vi "source_measure.vi"(8 "error in (no error)":errorcluster, 11 "Input parameters":T1={"Measurement type"=enum."Debug", "Sensor type"=enum."HPK_8in_271ch", "Identifier"="test.txt", "Open after execution?"=FALSE, "Plot after execution?"=FALSE, "Display channel"=0, "Voltage Delay (s)"=0.5, "Switch Delay (s)"=0.01, "VISA resource name source"="", "VISA resource name DMM"="", "VISA resource name LCR"="", "Compliance  Level (A)"=10.0, "Voltage Limit (V)"=1000.0, "Data storage location"="", "Scan voltages"="", "Use source as DMM?"=FALSE, "LCR signal frequenzy (Hz)"=10.0, "DMM device"=enum."Keithley2001", "Sampling number"=1, "Use env. sensors on"=enum."Sensirion sht1x/7x", "Switchboard Handle"=0, "Use Switchboard"=FALSE, "LCR signal voltage (V)"=10000.0, "Repeat"=1, "Scan voltages IV"="", "Scan voltages CV"="", "Hex pad numbers?"=FALSE, "Set measurement type"=enum."Debug", "Custom pad scan"="", "IV voltage Delay (s)"=0.5, "CV voltage Delay (s)"=0.5, "Needle measurement?"=FALSE, "Comments"="test.txt", "LCR signal frequenzy (kHz)"=10.0, "Compliance  Level (uA)"=10.0, "Open Correction Array"=array2304x3[6912 elements], "Current set voltage"=0.0, "Last set voltage"=0.0, "Current channel"=0, "Last OpenCorrection index"=-1, "Total curr/vltg every x steps"=10, "Current channel iteration"=0, "No CV corrections"=FALSE, "Mapfile"="", "Corrfile"="", "IV voltage file"=path "", "CV voltage file"=path "", "IV Switch Delay (s)"=0.01, "CV Switch Delay (s)"=0.01, "Invert polarity"=FALSE, "Set debug dirs"=FALSE, "Is n on p"=FALSE, "Source interlock?"=TRUE, "Voltage file used?"=FALSE, "Pad mask"="", "Mask pad above (uA)"=1.0, "LCR device"=enum."LCR_E4980", "Source device"=enum."Source_2410", "HexPlot binary path"="", "PadReductionFactor"=1.0, "Temperature degC"="", "Fluence [neq]"="", "Annealing [min]"=""} {"CV Switch Delay (s)" format="%#_13g"; "IV Switch Delay (s)" format="%#_13g"; "Last set voltage" format="%#_13g"; "Current set voltage" format="%#_13g"; "CV voltage Delay (s)" format="%#_13g"; "IV voltage Delay (s)" format="%#_13g"; "Voltage Limit (V)" format="%#_13g"; "Voltage Delay (s)" format="%#_13g"; "Switch Delay (s)" format="%#_13g"}) -> (0 "error out":errorcluster, 2 "Total current":dbl, 3 "Input parameters":T1={"Measurement type"=enum."Debug", "Sensor type"=enum."HPK_8in_271ch", "Identifier"="test.txt", "Open after execution?"=FALSE, "Plot after execution?"=FALSE, "Display channel"=0, "Voltage Delay (s)"=0.5, "Switch Delay (s)"=0.01, "VISA resource name source"="", "VISA resource name DMM"="", "VISA resource name LCR"="", "Compliance  Level (A)"=10.0, "Voltage Limit (V)"=1000.0, "Data storage location"="", "Scan voltages"="", "Use source as DMM?"=FALSE, "LCR signal frequenzy (Hz)"=10.0, "DMM device"=enum."Keithley2001", "Sampling number"=1, "Use env. sensors on"=enum."Sensirion sht1x/7x", "Switchboard Handle"=0, "Use Switchboard"=FALSE, "LCR signal voltage (V)"=10000.0, "Repeat"=1, "Scan voltages IV"="", "Scan voltages CV"="", "Hex pad numbers?"=FALSE, "Set measurement type"=enum."Debug", "Custom pad scan"="", "IV voltage Delay (s)"=0.5, "CV voltage Delay (s)"=0.5, "Needle measurement?"=FALSE, "Comments"="test.txt", "LCR signal frequenzy (kHz)"=10.0, "Compliance  Level (uA)"=10.0, "Open Correction Array"=array2304x3[6912 elements], "Current set voltage"=0.0, "Last set voltage"=0.0, "Current channel"=0, "Last OpenCorrection index"=-1, "Total curr/vltg every x steps"=10, "Current channel iteration"=0, "No CV corrections"=FALSE, "Mapfile"="", "Corrfile"="", "IV voltage file"=path "", "CV voltage file"=path "", "IV Switch Delay (s)"=0.01, "CV Switch Delay (s)"=0.01, "Invert polarity"=FALSE, "Set debug dirs"=FALSE, "Is n on p"=FALSE, "Source interlock?"=TRUE, "Voltage file used?"=FALSE, "Pad mask"="", "Mask pad above (uA)"=1.0, "LCR device"=enum."LCR_E4980", "Source device"=enum."Source_2410", "HexPlot binary path"="", "PadReductionFactor"=1.0, "Temperature degC"="", "Fluence [neq]"="", "Annealing [min]"=""} {"CV Switch Delay (s)" format="%#_13g"; "IV Switch Delay (s)" format="%#_13g"; "Last set voltage" format="%#_13g"; "Current set voltage" format="%#_13g"; "CV voltage Delay (s)" format="%#_13g"; "IV voltage Delay (s)" format="%#_13g"; "Voltage Limit (V)" format="%#_13g"; "Voltage Delay (s)" format="%#_13g"; "Switch Delay (s)" format="%#_13g"}, 4 "Compliance reached?":bool, 5 "Actual voltage":dbl)   [LabVIEW 2020]
doc: "Determines current voltage and current through source meter."
uses:
  <instrlib>/Keithley 24XX/Keithley 24XX.lvlib
  <instrlib>/Keithley 648X Series/Keithley 648X Series.lvlib
  input_params.ctl
panel:
  out "Effective resistance":sgl
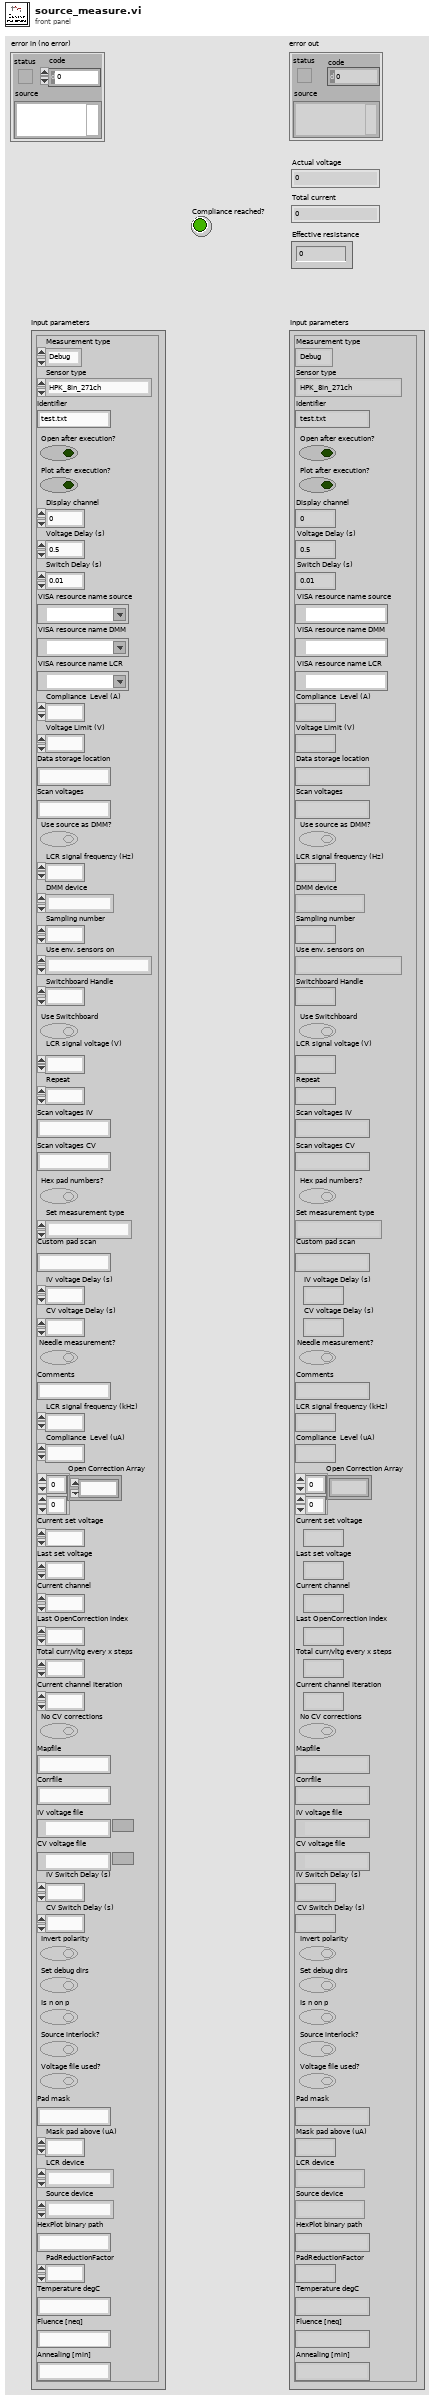
[diagram p1: front panel]
types:
  T1 = typedef "input_params.ctl" = cluster{"Measurement type":enum16{"IV", "CV", "Debug", "Test_contact"}, "Sensor type":enum16{"HPK_6in_135ch", "HPK_8in_271ch", "IFX_8in_256ch", "Diode", "HPK_6in_239ch", "Full_Matrix", "HPK_8in_271ch_full", "LumiCal", "HPK_8in_444ch", "HPK_8in_198ch_2019", "HPK_8in_MGW_LD_full", "HPK_8in_MGW_LD_a_type_top", "HPK_8in_MGW_LD_a_type_bottom", "HPK_8in_MGW_LD_b_type_left", "HPK_8in_MGW_LD_b_type_right", "HPK_8in_MGW_LD_c_type_left", "HPK_8in_MGW_LD_c_type_right", "HPK_8in_MGW_HD_full", "HPK_8in_MGW_HD_a_type_top", "HPK_8in_MGW_HD_a_type_bottom", "HPK_8in_MGW_HD_b_type_left", "HPK_8in_MGW_HD_b_type_right", "HPK_8in_MGW_HD_c_type_left", "HPK_8in_MGW_HD_c_type_right", "CALICE_6in_256ch"}, "Identifier":string, "Open after execution?":bool, "Plot after execution?":bool, "Display channel":i32, "Voltage Delay (s)":dbl, "Switch Delay (s)":dbl, "VISA resource name source":refnum<visa-resource-name>, "VISA resource name DMM":refnum<visa-resource-name>, "VISA resource name LCR":refnum<visa-resource-name>, "Compliance  Level (A)":dbl, "Voltage Limit (V)":dbl, "Data storage location":string, "Scan voltages":string, "Use source as DMM?":bool, "LCR signal frequenzy (Hz)":dbl, "DMM device":enum16{"Keithley2001", "Keithley2450", "Keithley2410", "Keithley6485", "Keithley6487", "Keithley6517"}, "Sampling number":i32, "Use env. sensors on":enum16{"Sensirion sht1x/7x", "Switch Matrix", "Probecard"}, "Switchboard Handle":u32, "Use Switchboard":bool, "LCR signal voltage (V)":dbl, "Repeat":i32, "Scan voltages IV":string, "Scan voltages CV":string, "Hex pad numbers?":bool, "Set measurement type":enum16{"IV", "CV", "Debug", "Test_contact", "IV+CV"}, "Custom pad scan":string, "IV voltage Delay (s)":dbl, "CV voltage Delay (s)":dbl, "Needle measurement?":bool, "Comments":string, "LCR signal frequenzy (kHz)":dbl, "Compliance  Level (uA)":dbl, "Open Correction Array":dbl[][], "Current set voltage":dbl, "Last set voltage":dbl, "Current channel":i32, "Last OpenCorrection index":i32, "Total curr/vltg every x steps":i32, "Current channel iteration":i32, "No CV corrections":bool, "Mapfile":string, "Corrfile":string, "IV voltage file":path, "CV voltage file":path, "IV Switch Delay (s)":dbl, "CV Switch Delay (s)":dbl, "Invert polarity":bool, "Set debug dirs":bool, "Is n on p":bool, "Source interlock?":bool, "Voltage file used?":bool, "Pad mask":string, "Mask pad above (uA)":dbl, "LCR device":enum16{"LCR_E4980", "AGILENT_4263X"}, "Source device":enum16{"Source_2410", "Source_6487"}, "HexPlot binary path":string, "PadReductionFactor":dbl, "Temperature degC":string, "Fluence [neq]":string, "Annealing [min]":string}
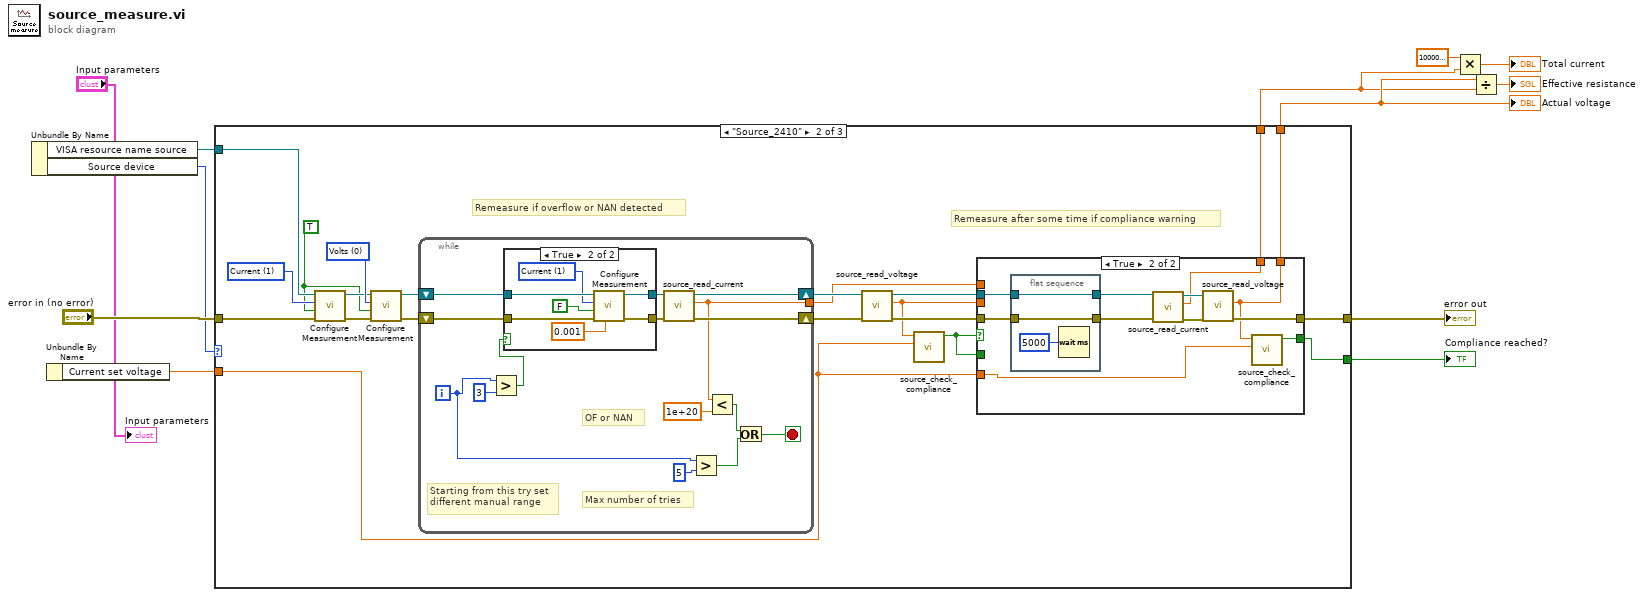
[diagram p0: block diagram]
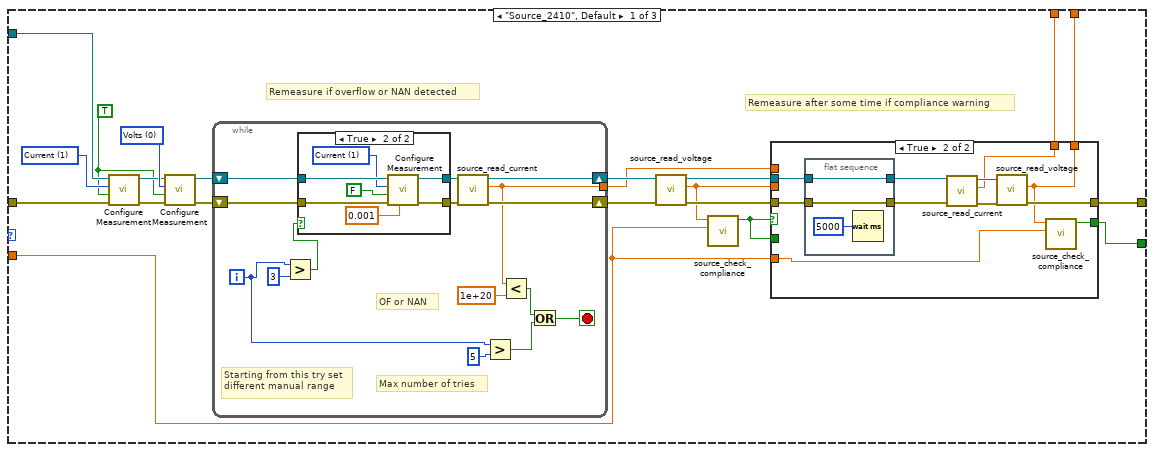
[diagram p2: hidden frame]
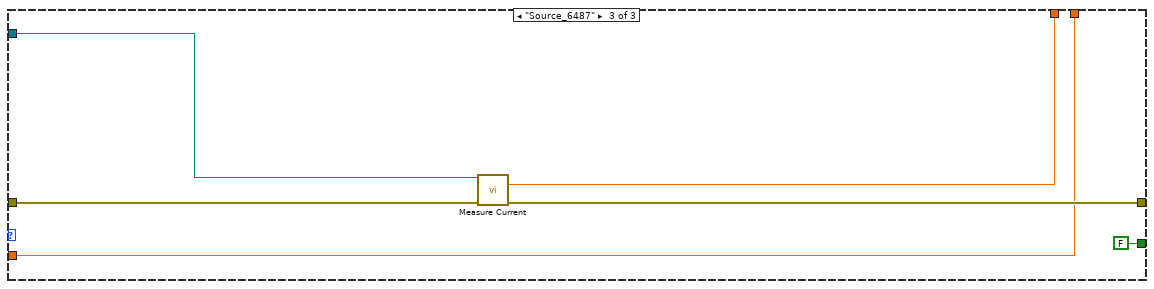
[diagram p7: hidden frame]
diagram:
  n1 = Unbundle By Name("Input parameters") -> ("VISA resource name source"=w12:refnum<visa-resource-name>, "Source device"=w1:enum16{"Source_2410", "Source_6487"})
  n2 = Unbundle By Name("Input parameters") -> ("Current set voltage"=w2:dbl)
  n3 = case shown="\"Source_2470\"" w1 {
    tunnel: w12 -> [w33 w96 w140]
    tunnel: "error in (no error)" -> [w32 w95 w139]
    tunnel: [w21 w84 w143] -> w6
    tunnel: [w19 w82 FALSE ("Is compliance?")] -> w5
    tunnel: [w17 w80 w141] -> w4
    tunnel: [w16 w79 w142] -> w3
    tunnel: w2 -> [w14 w77 w141]
    frame "Source_2410", Default {
      w27 = TRUE
      w30 = u16 0 items=["Volts", "Current", "Resistance"] ("Function (0: Volts)")
      w31 = u16 1 items=["Volts", "Current", "Resistance"] ("Function (0: Volts)")
      # "Remeasure after some time if compliance warning"
      # "Remeasure if overflow or NAN detected"
      n4 = call <instrlib>:"Configure Measurement.vi"("error in (no error)"=w32, "Enable Auto Range (T:Enable)"=w27, "Function (0: Volts)"=w31, "VISA resource name"=w33) -> ("error out"=w29:errorcluster, "VISA resource name out"=w28:refnum<visa-resource-name>)  [unwired: 6 in]
      n5 = call <instrlib>:"Configure Measurement.vi"("error in (no error)"=w29, "Enable Auto Range (T:Enable)"=w27, "Function (0: Volts)"=w30, "VISA resource name"=w28) -> ("error out"=w26:errorcluster, "VISA resource name out"=w25:refnum<visa-resource-name>)  [unwired: 6 in]
      n6 = while {
        tunnel: [w44] -> w13
        shift-right: [w48] -> w24
        shift-left: w26 -> [w38]
        shift-right: [w47] -> w23
        shift-left: w25 -> [w36]
        i -> [w40]
        stop <- w41 stop-if-true
        # "Starting from this try set\ndifferent manual range"
        # "OF or NAN"
        # "Max number of tries"
        n7 = Greater?(x=w40, y=3) -> (0:w34:bool)
        n8 = case shown="True" w34 {
          tunnel: w38 -> [w49 w57]
          tunnel: [w49 w56] -> w37
          tunnel: w36 -> [w50 w55]
          tunnel: [w50 w54] -> w35
          frame False {
          }
          frame True {
            w53 = u16 1 items=["Volts", "Current", "Resistance"] ("Function (0: Volts)")
            n9 = call <instrlib>:"Configure Measurement.vi"("Manual Range (1.0)"=0.001, "error in (no error)"=w57, "Enable Auto Range (T:Enable)"=FALSE, "Function (0: Volts)"=w53, "VISA resource name"=w55) -> ("error out"=w56:errorcluster, "VISA resource name out"=w54:refnum<visa-resource-name>)  [unwired: 5 in]
          }
        }
        n10 = call "source_read_current.vi"("error in (no error)"=w37, "VISA resource name"=w35) -> ("error out"=w48:errorcluster, "Value"=w44:sgl, "VISA resource name out"=w47:refnum<visa-resource-name>)  [unwired: 7 in]
        n11 = Greater?(x=w40, y=5) -> (0:w42:bool)
        n12 = Less?(x=w44, y=1e+20) -> (x < y?=w43:bool)
        n13 = Or(x=w43, y=w42) -> (x .or. y?=w41:bool)
      }
      n14 = call "source_read_voltage.vi"("error in (no error)"=w24, "VISA resource name"=w23) -> ("error out"=w22:errorcluster, "Value"=w18:sgl, "VISA resource name out"=w15:refnum<visa-resource-name>)  [unwired: 7 in]
      n15 = call "source_check_compliance.vi"("Target voltage"=w14, "Actual voltage"=w18) -> ("Is compliance?"=w20:bool)  [unwired: 9 in]
      n16 = case shown="True" w20 {
        tunnel: w22 -> [w61 w68]
        tunnel: [w61 w72] -> w21
        tunnel: w20 -> [w60 _]
        tunnel: [w60 w70] -> w19
        tunnel: w18 -> [w59 _]
        tunnel: w13 -> [w58 _]
        tunnel: [w59 w67] -> w17
        tunnel: [w58 w62] -> w16
        tunnel: w15 -> [_ w69]
        tunnel: w14 -> [_ w71]
        frame False {
        }
        frame True {
          n17 = flat-sequence {
            tunnel: w69 -> [w73]
            tunnel: w68 -> [w74]
            tunnel: [w74] -> w66
            tunnel: [w73] -> w64
            frame #0 {
              n18 = Wait (ms)(milliseconds to wait=u32 5000) -> ()  [unwired: 1 out]
            }
          }
          n19 = call "source_read_current.vi"("error in (no error)"=w66, "VISA resource name"=w64) -> ("error out"=w65:errorcluster, "Value"=w62:sgl, "VISA resource name out"=w63:refnum<visa-resource-name>)  [unwired: 7 in]
          n20 = call "source_read_voltage.vi"("error in (no error)"=w65, "VISA resource name"=w63) -> ("error out"=w72:errorcluster, "Value"=w67:sgl)  [unwired: 7 in, 1 out]
          n21 = call "source_check_compliance.vi"("Target voltage"=w71, "Actual voltage"=w67) -> ("Is compliance?"=w70:bool)  [unwired: 9 in]
        }
      }
    }
    frame "Source_2410" {
      w90 = TRUE
      w93 = u16 0 items=["Volts", "Current", "Resistance"] ("Function (0: Volts)")
      w94 = u16 1 items=["Volts", "Current", "Resistance"] ("Function (0: Volts)")
      # "Remeasure after some time if compliance warning"
      # "Remeasure if overflow or NAN detected"
      n22 = call <instrlib>:"Configure Measurement.vi"("error in (no error)"=w95, "Enable Auto Range (T:Enable)"=w90, "Function (0: Volts)"=w94, "VISA resource name"=w96) -> ("error out"=w92:errorcluster, "VISA resource name out"=w91:refnum<visa-resource-name>)  [unwired: 6 in]
      n23 = call <instrlib>:"Configure Measurement.vi"("error in (no error)"=w92, "Enable Auto Range (T:Enable)"=w90, "Function (0: Volts)"=w93, "VISA resource name"=w91) -> ("error out"=w89:errorcluster, "VISA resource name out"=w88:refnum<visa-resource-name>)  [unwired: 6 in]
      n24 = while {
        tunnel: [w107] -> w76
        shift-right: [w111] -> w87
        shift-left: w89 -> [w101]
        shift-right: [w110] -> w86
        shift-left: w88 -> [w99]
        i -> [w103]
        stop <- w104 stop-if-true
        # "Starting from this try set\ndifferent manual range"
        # "OF or NAN"
        # "Max number of tries"
        n25 = Greater?(x=w103, y=3) -> (0:w97:bool)
        n26 = case shown="True" w97 {
          tunnel: w101 -> [w112 w120]
          tunnel: [w112 w119] -> w100
          tunnel: w99 -> [w113 w118]
          tunnel: [w113 w117] -> w98
          frame False {
          }
          frame True {
            w116 = u16 1 items=["Volts", "Current", "Resistance"] ("Function (0: Volts)")
            n27 = call <instrlib>:"Configure Measurement.vi"("Manual Range (1.0)"=0.001, "error in (no error)"=w120, "Enable Auto Range (T:Enable)"=FALSE, "Function (0: Volts)"=w116, "VISA resource name"=w118) -> ("error out"=w119:errorcluster, "VISA resource name out"=w117:refnum<visa-resource-name>)  [unwired: 5 in]
          }
        }
        n28 = call "source_read_current.vi"("error in (no error)"=w100, "VISA resource name"=w98) -> ("error out"=w111:errorcluster, "Value"=w107:sgl, "VISA resource name out"=w110:refnum<visa-resource-name>)  [unwired: 7 in]
        n29 = Greater?(x=w103, y=5) -> (0:w105:bool)
        n30 = Less?(x=w107, y=1e+20) -> (x < y?=w106:bool)
        n31 = Or(x=w106, y=w105) -> (x .or. y?=w104:bool)
      }
      n32 = call "source_read_voltage.vi"("error in (no error)"=w87, "VISA resource name"=w86) -> ("error out"=w85:errorcluster, "Value"=w81:sgl, "VISA resource name out"=w78:refnum<visa-resource-name>)  [unwired: 7 in]
      n33 = call "source_check_compliance.vi"("Target voltage"=w77, "Actual voltage"=w81) -> ("Is compliance?"=w83:bool)  [unwired: 9 in]
      n34 = case shown="True" w83 {
        tunnel: w85 -> [w124 w131]
        tunnel: [w124 w135] -> w84
        tunnel: w83 -> [w123 _]
        tunnel: [w123 w133] -> w82
        tunnel: w81 -> [w122 _]
        tunnel: w76 -> [w121 _]
        tunnel: [w122 w130] -> w80
        tunnel: [w121 w125] -> w79
        tunnel: w78 -> [_ w132]
        tunnel: w77 -> [_ w134]
        frame False {
        }
        frame True {
          n35 = flat-sequence {
            tunnel: w132 -> [w136]
            tunnel: w131 -> [w137]
            tunnel: [w137] -> w129
            tunnel: [w136] -> w127
            frame #0 {
              n36 = Wait (ms)(milliseconds to wait=u32 5000) -> ()  [unwired: 1 out]
            }
          }
          n37 = call "source_read_current.vi"("error in (no error)"=w129, "VISA resource name"=w127) -> ("error out"=w128:errorcluster, "Value"=w125:sgl, "VISA resource name out"=w126:refnum<visa-resource-name>)  [unwired: 7 in]
          n38 = call "source_read_voltage.vi"("error in (no error)"=w128, "VISA resource name"=w126) -> ("error out"=w135:errorcluster, "Value"=w130:sgl)  [unwired: 7 in, 1 out]
          n39 = call "source_check_compliance.vi"("Target voltage"=w134, "Actual voltage"=w130) -> ("Is compliance?"=w133:bool)  [unwired: 9 in]
        }
      }
    }
    frame "Source_6487" {
      n40 = call <instrlib>:"Measure Current.vi"("VISA resource name"=w140, "error in (no error)"=w139) -> ("Measurement"=w142:dbl, "error out"=w143:errorcluster)  [unwired: 11 in, 1 out]
    }
  }
  "Actual voltage" <- w4
  "error out" <- w6
  "Compliance reached?" <- w5
  n41 = Multiply(x=sgl 1000000000.0 ("Value"), y=w3) -> (x*y=→"Total current":dbl)
  n42 = Divide(x=w4, y=w3) -> (x/y=→"Effective resistance":dbl)
  "Input parameters" <- "Input parameters"
